vi "Start Motion.vi"(8 "error in (no error)":errorcluster, 11 "Motion In":refnum<class "BasicTerminalBinding.lvclass">) -> (0 "error out":errorcluster, 3 "Motion Out":refnum<class "BasicTerminalBinding.lvclass">)   [LabVIEW 2017, in "TestViewables.lvlib" / "BasicTerminalBinding.lvclass"]
uses:
  BasicTerminalBinding.lvclass
  C:/Program Files (x86)/National Instruments/LabVIEW 2017/vi.lib/ActorFramework/Actor/Actor.lvclass
  <vilib>/ActorFramework/Message Enqueuer/Message Priority.ctl
  gpm_packages/@cs/actor-framework-messages/Source/MessageCycle/Message Cycle Notifications.ctl
  BasicTerminalBinding Messages/Check If Done Msg/Check If Done Msg.lvclass
  C:/Program Files (x86)/National Instruments/LabVIEW 2017/vi.lib/ActorFramework/Message/Message.lvclass
  Send Warning Folder/Send Warning.lvclass
  <vilib>/ActorFramework/Actor/Actor.lvclass/Actor.ctl
  <vilib>/ActorFramework/Message Enqueuer/Message Enqueuer.lvclass/Message Enqueuer.ctl
  gpm_packages/@cs/actor-framework-messages/Source/MessageCycle/MessageCycle.lvclass/MessageCycle.ctl
  <vilib>/ActorFramework/Message Enqueuer/Init from Existing Queue.vi
  <vilib>/ActorFramework/Message Enqueuer/Enqueue.vi
  gpm_packages/@cs/actor-framework-messages/Source/MessageCycle/MessageCycle.lvclass
  gpm_packages/@cs/actor-framework-messages/Source/MessageCycle/Launch Deferred Timeout Notifier.vi
  <vilib>/ActorFramework/Message Priority Queue/Priority Enqueue.vi
  <vilib>/ActorFramework/Message Enqueuer/Message Enqueuer.lvclass
  <vilib>/ActorFramework/Actor/Actor.lvclass
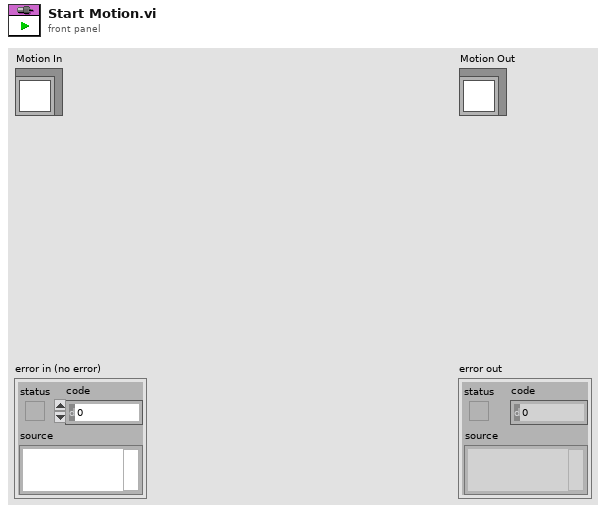
[diagram p1: front panel]
types:
  T1 = typedef "MessageCycle.lvclass/Message Cycle Notifications.ctl" = enum16{"Process Final Copy and Stop", "Stop Immediately", "Substitute Last Message and Stop"}
  T2 = typedef "Actor Framework.lvlib/Message Enqueuer.lvclass/Message Priority.ctl" = enum16{"Low", "Normal", "High"}
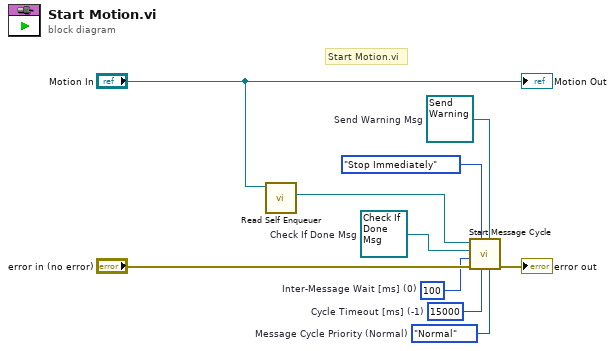
[diagram p0: block diagram]
diagram:
  w1 = refnum<class "Send Warning.lvclass"> refnum  # Send Warning Msg
  w2 = refnum<class "Check If Done Msg.lvclass"> refnum  # Check If Done Msg
  w4 = Message_Priority."Normal"  # Message Cycle Priority (Normal)
  w5 = 15000  # Cycle Timeout [ms] (-1)
  w6 = 100  # Inter-Message Wait [ms] (0)
  # "Start Motion.vi"
  n1 = call <vilib>:"Read Self Enqueuer.vi"("Actor"="Motion In") -> ("Self Enqueuer"=w7:refnum<class "Message Enqueuer.lvclass">)  [unwired: 10 in]
  n2 = call "Start Message Cycle.vi"("Message Cycle Priority (Normal)"=w4, "Last Message"=w1, "Cycle Timeout [ms] (-1)"=w5, "Timeout Action"=Message_Cycle_Notifications."Stop Immediately", "error in (no error)"="error in (no error)", "Inter-Message Wait [ms] (0)"=w6, "Message"=w2, "Message Enqueuer"=w7) -> ("error out"=→"error out":errorcluster)  [unwired: 1 in, 2 out]
  "Motion Out" <- "Motion In"
